vi "links.get.vi"(8 "error in (no error)":errorcluster, 11 "Run in":refnum<class "Run.lvclass">) -> (0 "error out":errorcluster, 2 "links":cluster{"url":string, "title":string}[](array[cluster]), 3 "Run out":refnum<class "Run.lvclass">)   [LabVIEW 2020, in "Run.lvclass"]
uses:
  Run.lvclass
  Run.lvclass/Run.ctl
  5b00825a-b8ea-4fac-8dbd-770dc6ccb513.vi
  5b00825a-b8ea-4fac-8dbd-770dc6ccb513.vi/32c3acc2-0975-485a-8283-62feb0f3dc4f.vi
  run_properties.get.vi
  <vilib>/JDP Science/JSONtext/JSON type.vi
  <vilib>/JDP Science/JSONtext/JSON text to Variant.vi
  <vilib>/JDP Science/JSONtext/LVClass Serializer/JSONtext LVClass Serializer.lvclass
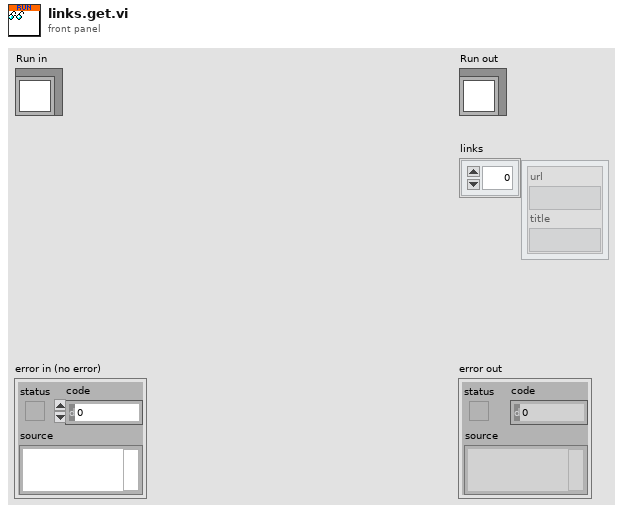
[diagram p1: front panel]
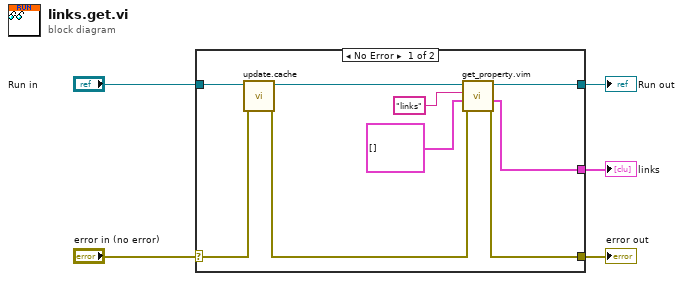
[diagram p0: block diagram]
diagram:
  n1 = case shown="No Error" "error in (no error)" {
    selector: "error in (no error)" -> [w14 w15]
    tunnel: [w9 w15] -> w4
    tunnel: [w10 w16] -> w2
    tunnel: "Run in" -> [w13 w16]
    tunnel: [w6 _] -> w1
    frame No Error {
      n2 = call "update.cache.vi"("error in"=w14, "Run in"=w13) -> ("error out"=w11:errorcluster, "Run out"=w12:refnum<class "Run.lvclass">)  [unwired: 8 in]
      n3 = call "get_property.vim"("error in"=w11, "default value and type"=cluster{"url":string, "title":string}[] [] ("links"), "Property Name"="links", "Run in"=w12) -> ("error out"=w9:errorcluster, "Value"=w6:cluster{"url":string, "title":string}[], "Run out"=w10:refnum<class "Run.lvclass">)  [unwired: 5 in]
    }
    frame Error {
    }
  }
  "error out" <- w4
  "Run out" <- w2
  "links" <- w1
